vi "Get Readout Modes.vi"(8 "error in (no error)":errorcluster, 11 "Photometrics Camera in":refnum<class "Photometrics Camera.lvclass">) -> (0 "error out":errorcluster, 3 "Photometrics Camera out":refnum<class "Photometrics Camera.lvclass">)   [LabVIEW 2023, in "Photometrics Camera.lvlib" / "Photometrics Camera.lvclass"]
uses:
  Photometrics Camera.lvclass
  C:/Program Files/National Instruments/LabVIEW 2023/vi.lib/ActorFramework/Actor/Actor.lvclass
  Public/Documents/Photometrics/TPM-LabVIEWSamples BETA/TPM LabVIEW adapter/Camera/Camera.lvclass
  <vilib>/ActorFramework/Actor/Actor.lvclass/Actor.ctl
  Application Messages/Update Camera Modes Msg/Update Camera Modes Msg.lvclass/Update Camera Modes Msg.ctl
  <vilib>/ActorFramework/Message Enqueuer/Message Enqueuer.lvclass/Message Enqueuer.ctl
  <vilib>/ActorFramework/Message Enqueuer/Enqueue.vi
  Application Messages/Update Camera Modes Msg/Update Camera Modes Msg.lvclass
  C:/Program Files/National Instruments/LabVIEW 2023/vi.lib/ActorFramework/Message/Message.lvclass
  <vilib>/ActorFramework/Message Priority Queue/Priority Enqueue.vi
  <vilib>/ActorFramework/Actor/Actor.lvclass
panel:
  out "StringsAndValues":cluster{"String":string, "Value":i32}[](array[cluster])
  in  "Gain":string(combo)
  in  "Readout Ports/Speeds":string(combo)
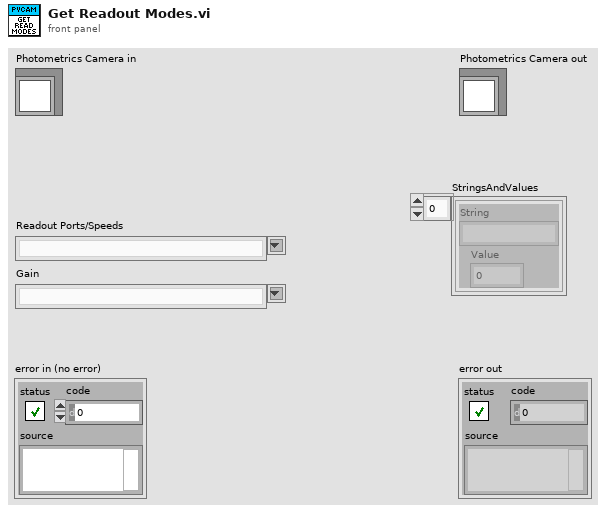
[diagram p1: front panel]
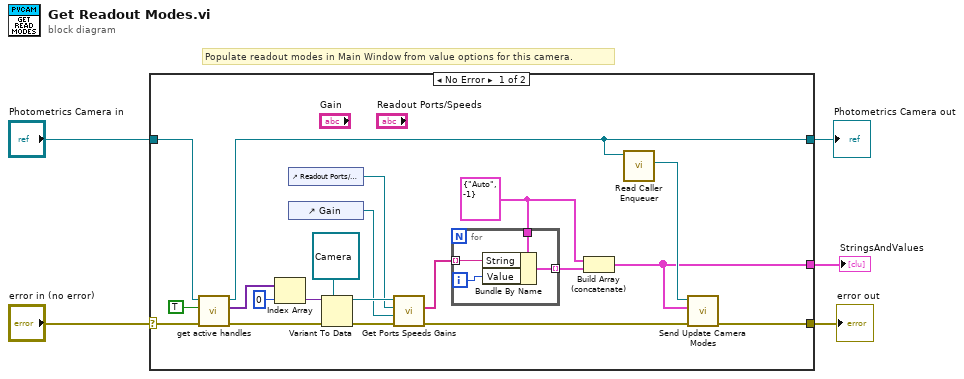
[diagram p0: block diagram]
diagram:
  # "Populate readout modes in Main Window from value options for this camera."
  n1 = case shown="No Error" "error in (no error)" {
    selector: "error in (no error)" -> [w25 w31]
    tunnel: [w6 w31] -> w4
    tunnel: [w10 w30] -> w2
    tunnel: "Photometrics Camera in" -> [w23 w30]
    tunnel: [w8 _] -> w1
    frame No Error {
      w11 = cluster{"String":string, "Value":i32} {"String"="Auto", "Value"=-1}
      n2 = call-dynamic "get active handles.vi"("error in (no error)"=w25, "Return All?"=TRUE, "Camera in"=w23) -> ("error out"=w19:errorcluster, "Handles"=w20:variant[], "Camera out"=w10:refnum<class "Photometrics Camera.lvclass">)  [unwired: 4 in, 2 out]
      n3 = Index Array(array=w20, index=0) -> (element=w18:variant)
      n4 = control-ref of="Readout Ports/Speeds"() -> (w15:refnum<vi>)
      n5 = control-ref of="Gain"() -> (w14:refnum<vi>)
      n6 = Variant To Data(error in=w19, type=refnum<class "Camera.lvclass"> refnum ("Camera In"), Variant=w18) -> (data=w16:refnum<class "Camera.lvclass">, error out=w17:errorcluster)
      n7 = call "Get Ports Speeds Gains.vi"("error in (no error)"=w17, "Gains cbx"=w14, "Ports and Speeds cbx"=w15, "Camera In"=w16) -> ("error out"=w7:errorcluster, "Port/Speed Options"=w13:string[])  [unwired: 4 in, 2 out]
      n8 = for {
        tunnel: w13 -> [w29] mode=indexing
        tunnel: w11 -> [w28]
        tunnel: [w26] -> w12 mode=indexing
        i -> [w27]
        n9 = Bundle By Name(cluster=w28, "String"=w29, "Value"=w27) -> (w26:cluster{"String":string, "Value":i32})
      }
      n10 = Build Array (concatenate)(w11, w12) -> (w8:cluster{"String":string, "Value":i32}[])
      n11 = call <vilib>:"Read Caller Enqueuer.vi"("Actor"=w10) -> ("Caller Enqueuer"=w9:refnum<class "Message Enqueuer.lvclass">)  [unwired: 10 in]
      n12 = call "Send Update Camera Modes.vi"("error in (no error)"=w7, "StringsAndValues"=w8, "Message Enqueuer"=w9) -> ("error out"=w6:errorcluster)  [unwired: 7 in, 1 out]
    }
    frame Error {
    }
  }
  "error out" <- w4
  "Photometrics Camera out" <- w2
  "StringsAndValues" <- w1
